vi "Read Encoders.vi"(8 "Reset":bool) -> (3 "Encoder Data":T1 {"Omni"."Ticks" format="%#.6g"; "Right"."Ticks" format="%#.6g"; "Left"."Ticks" format="%#.6g"})   [LabVIEW 2013]
uses:
  Encoder Data.ctl
  Single Encoder Data.ctl
  Robot Global Data.vi
  <vilib>/addons/control/pid/pid.llb/PID Control Input Filter.vi
  <vilib>/addons/control/pid/pid.llb/PID Control Input Filter (DBL).vi
  <vilib>/Rock Robotics/WPI/Encoder/WPI_EncoderGet.vi
  <vilib>/Rock Robotics/WPI/Encoder/WPI_EncoderReset.vi
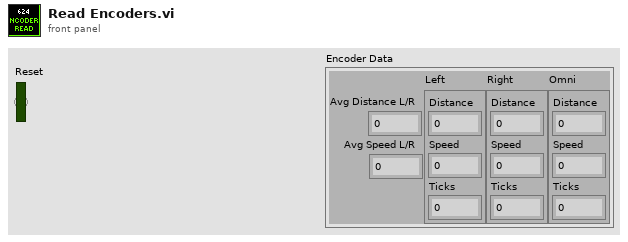
[diagram p1: front panel]
types:
  T1 = typedef "Encoder Data.ctl" = cluster{"Avg Distance L/R":dbl, "Avg Speed L/R":dbl, "Left":T2, "Right":T2, "Omni":T2}
  T2 = typedef "Single Encoder Data.ctl" = cluster{"Distance":dbl, "Speed":dbl, "Ticks":dbl}
  T3 = typedef "Dashboard UDP Packet.ctl" = cluster{"Camera":T4, "Gyro":T5, "Encoder":T7, "Auto Shift":T8, "Auton":T9, "Drive/Ramp X":dbl, "Drive/Ramp Y":dbl, "Drive/Battery Cutoff":dbl, "Pressure/Compressor Min Voltage":dbl, "Pressure/Compressor Delay":dbl, "Controller/Strafe Correction":bool, "Shooter":T10, "Rollers":T11, "Abort":bool, "Finish":bool, "Halo Time":dbl}
  T4 = typedef "Camera Controls.ctl" = cluster{"Camera/View Angle X":dbl, "Camera/Goal Track Timeout":dbl, "Camera/View Angle Y":dbl, "Camera/Goal Exposure":dbl, "Camera/Vision Receive Timeout":dbl, "Camera/Offset 1":dbl, "Camera/Offset 2":dbl}
  T5 = typedef "Gyro Controls.ctl" = cluster{"Gyro/Angle Tolerance":dbl, "Gyro/Steer Closeness Threshold":dbl, "Steer PID":T6, "Steer Close PID":T6}
  T6 = typedef "PID Params.ctl" = cluster{"max":dbl, "min":dbl, "P":dbl, "I":dbl, "D":dbl}
  T7 = typedef "Encoder Controls.ctl" = cluster{"Encoders/Reset":bool, "Encoders/Omni Constant":dbl, "Encoders/Omni Tick Constant":dbl, "Encoders/Left Constant":dbl, "Encoders/Right Constant":dbl, "Encoders/Right Tick Constant":dbl}
  T8 = typedef "Auto Shift Controls.ctl" = cluster{"AutoShift/Upshift Throttle Accel":dbl, "AutoShift/Speed Threshold":dbl, "AutoShift/Upshift Throttle":dbl, "AutoShift/Upshift Accel":dbl, "AutoShift/Downshift Accel":dbl, "AutoShift/Downshift Throttle":dbl, "AutoShift/Delay":dbl, "AutoShift/Enabled":bool}
  T9 = typedef "Auton Controls.ctl" = cluster{"Auton/Left Shoot X-Coord":dbl, "Auton/Right Shoot X-Coord":dbl, "DistDrive/Distance Stop Threshold":dbl, "DistDrive/Max Stop Speed":dbl, "Auton/Back Piston Time":dbl, "Auton/Manual Hot":bool, "Auton/Manual Hot Right":bool, "Default X PID":T6, "Default Y PID":T6}
  T10 = typedef "Shooter Controls.ctl" = cluster{"Shooter/Reset Time":dbl, "Shooter/Release Delay":dbl, "Shooter/Pressure Steady Time":dbl, "Shooter/Misfire Delay":dbl, "Shooter/Ball Settle Time":dbl, "Shooter/Line IR Delay":dbl, "Pressure/Upper PSI Time":dbl, "Pressure/Lower PSI Time":dbl, "Shooter/Punch Delay":dbl, "Shooter/Target Pressure":dbl, "Pressure/Line B":dbl, "Pressure/Line M":dbl, "Pressure/Shooter M":dbl, "Pressure/Shooter B":dbl}
  T11 = typedef "Roller Controls.ctl" = cluster{"Roller/Load IRs Verify Time":dbl, "Roller/Center IR Latch Time":dbl, "Roller/Speed Front":dbl, "Roller/Speed Back":dbl, "Roller/Entry Timeout":dbl, "Roller/To Center Timeout":dbl, "Roller/Sustain Time":dbl, "Roller/Verify Center Time":dbl}
  T12 = typedef "WPI_EncoderDevRef.ctl" = cluster{"DevStatus":errorcluster, "EncoderIndex":T13, "CounterIndex":T14, "DistancePerCount":dbl, "Decoding Type":T15}
  T13 = typedef "FPGA_EncoderIdx.ctl" = enum8{"Enc 0", "Enc 1", "Enc 2", "Enc 3", "Invalid"}
  T14 = typedef "FPGA_CounterCtrSystemIndex.ctl" = enum8{"Ctr 0", "Ctr 1", "Ctr 2", "Ctr 3", "Ctr 4", "Ctr 5", "Ctr 6", "Ctr 7", "Invalid"}
  T15 = typedef "WPI_EncoderType.ctl" = enum16{"1x", "2x", "4x"}
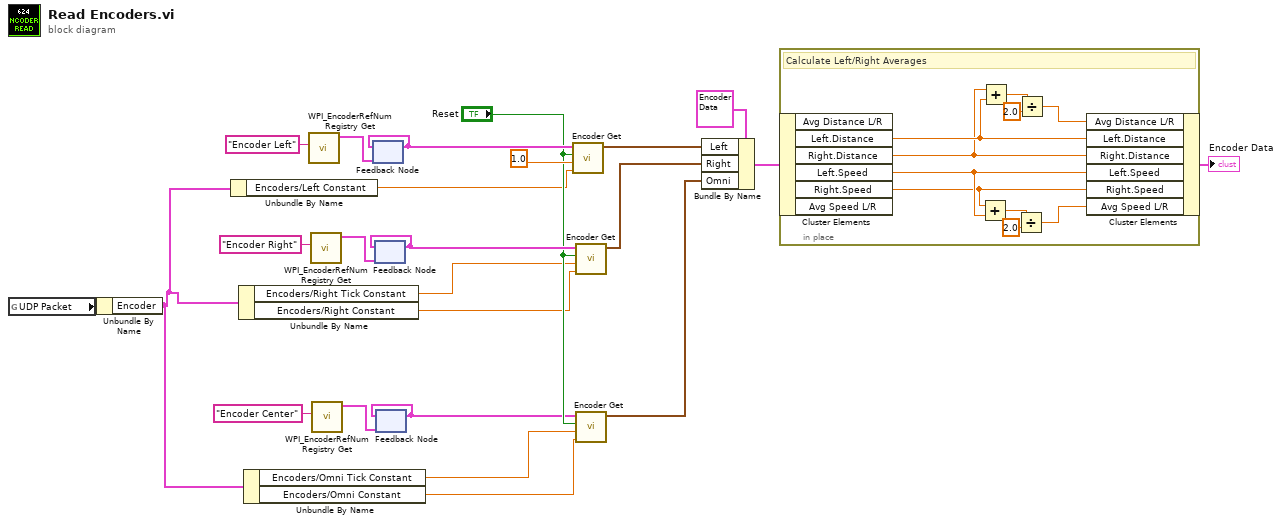
[diagram p0: block diagram]
diagram:
  n1 = global read "Robot Global Data.vi" "UDP Packet"() -> (w11:T3)
  n2 = Unbundle By Name(w11) -> ("Encoder"=w4:T7)
  n3 = Unbundle By Name(w4) -> ("Encoders/Left Constant"=w10:dbl)
  n4 = Unbundle By Name(w4) -> ("Encoders/Right Tick Constant"=w9:dbl, "Encoders/Right Constant"=w8:dbl)
  n5 = Unbundle By Name(w4) -> ("Encoders/Omni Tick Constant"=w3:dbl, "Encoders/Omni Constant"=w2:dbl)
  n6 = call <vilib>:"WPI_EncoderRefNum Registry Get.vi"("refnum name"="Encoder Left") -> ("EncoderDevRef"=w23:T12)  [unwired: 9 in, 1 out]
  n7 = call <vilib>:"WPI_EncoderRefNum Registry Get.vi"("refnum name"="Encoder Right") -> ("EncoderDevRef"=w18:T12)  [unwired: 9 in, 1 out]
  n8 = call <vilib>:"WPI_EncoderRefNum Registry Get.vi"("refnum name"="Encoder Center") -> ("EncoderDevRef"=w6:T12)  [unwired: 9 in, 1 out]
  n9 = feedback #1(w23) -> (w22:T12)
  n10 = feedback-in #1(w22) -> ()
  n11 = feedback #2(w18) -> (w19:T12)
  n12 = feedback-in #2(w19) -> ()
  n13 = feedback #3(w6) -> (w5:T12)
  n14 = feedback-in #3(w5) -> ()
  n15 = call "Encoder Get.vi"("Feet Constant"=w10, "Tick Constant"=1.0, "Reset"="Reset", "EncoderDevRef"=w22) -> ("Encoder Data"=w13:T2)  [unwired: 7 in]
  n16 = call "Encoder Get.vi"("Feet Constant"=w8, "Tick Constant"=w9, "Reset"="Reset", "EncoderDevRef"=w19) -> ("Encoder Data"=w15:T2)  [unwired: 7 in]
  n17 = call "Encoder Get.vi"("Feet Constant"=w2, "Tick Constant"=w3, "Reset"="Reset", "EncoderDevRef"=w5) -> ("Encoder Data"=w14:T2)  [unwired: 7 in]
  n18 = Bundle By Name(cluster=T1 {"Avg Distance L/R"=0.0, "Avg Speed L/R"=0.0, "Left"={"Distance"=0.0, "Speed"=0.0, "Ticks"=0.0}, "Right"={"Distance"=0.0, "Speed"=0.0, "Ticks"=0.0}, "Omni"={"Distance"=0.0, "Speed"=0.0, "Ticks"=0.0}} ("Encoder Data"), "Left"=w13, "Right"=w15, "Omni"=w14) -> (w12:T1)
  n19 = in-place {
    # "Calculate Left/Right Averages"
    n20 = in-place-cluster #4(w12) -> ("Left.Distance"=w29:dbl, "Right.Distance"=w28:dbl, "Left.Speed"=w27:dbl, "Right.Speed"=w26:dbl)  [unwired: 2 out]
    n21 = Add(x=w26, y=w27) -> (x+y=w31:dbl)
    n22 = Add(x=w28, y=w29) -> (x+y=w34:dbl)
    n23 = Divide(x=w31, y=2.0) -> (x/y=w25:dbl)
    n24 = Divide(x=w34, y=2.0) -> (x/y=w30:dbl)
    n25 = in-place-cluster #4("Avg Distance L/R"=w30, "Left.Distance"=w29, "Right.Distance"=w28, "Left.Speed"=w27, "Right.Speed"=w26, "Avg Speed L/R"=w25) -> (→"Encoder Data":T1)
  }
